vi "testBlockDMA_GERM.vi"(8 "error in (no error)":errorcluster, 11 "TestCase in":refnum<class "DSF CD GE Reflective Memory System Tests.lvclass">) -> (0 "error out":errorcluster, 3 "TestCase out":refnum<class "DSF CD GE Reflective Memory System Tests.lvclass">)   [LabVIEW 2019, in "DSF CD GE Reflective Memory System Tests.lvclass"]
uses:
  DSF CD GE Reflective Memory System Tests.lvclass
  C:/Program Files (x86)/National Instruments/LabVIEW 2019/vi.lib/addons/_JKI Toolkits/VI Tester/TestCase.llb/TestCase.lvclass
  niveristand-data-sharing-framework-custom-device-plugins/Components/Transceivers/GE Reflective Memory/Driver/Source/Typedefs/GE 5565PIORC.Typedef.DMA Wait Mode.ctl
  niveristand-data-sharing-framework-custom-device-plugins/Components/Transceivers/GE Reflective Memory/Driver/Source/GE 5565PIORC.lvclass
  <vilib>/addons/_JKI Toolkits/VI Tester/TestCase.llb/TestCase.lvclass
  fe7e187c-5126-4982-8e63-bd07b26320cd.vi
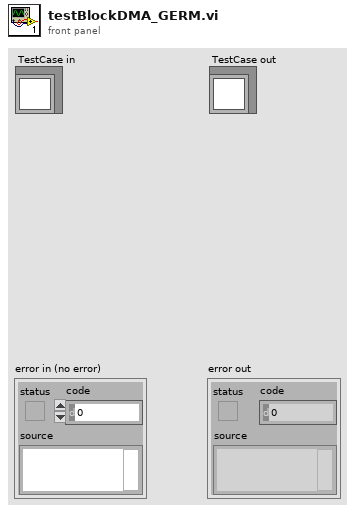
[diagram p1: front panel]
types:
  T1 = typedef "GE 5565PIORC.lvclass/GE 5565PIORC.Typedef.DMA Wait Mode.ctl" = enum16{"Polling", "Interrupt"}
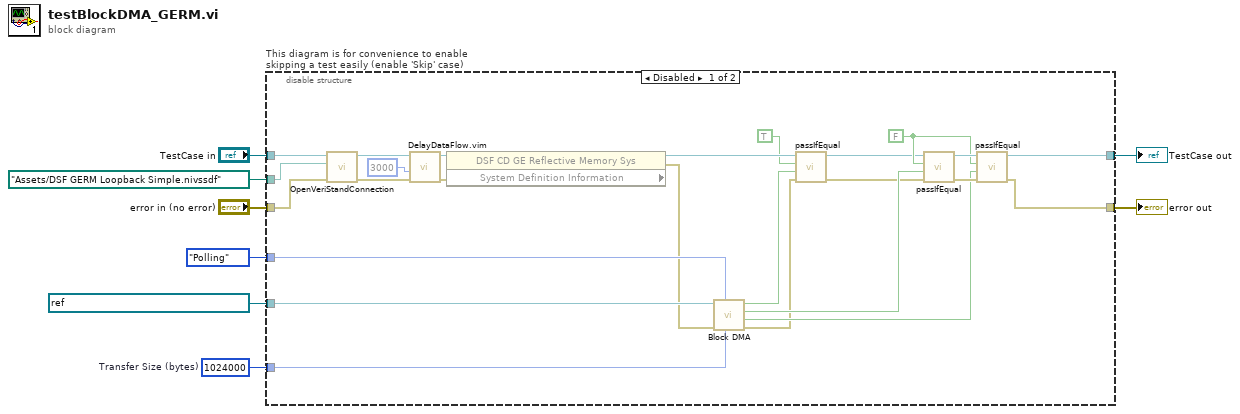
[diagram p0: block diagram]
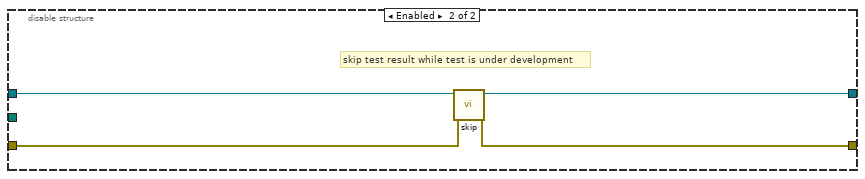
[diagram p2: hidden frame]
diagram:
  w2 = u32 1024000  # Transfer Size (bytes)
  n1 = disable-structure "This diagram is for convenience to enable skipping a test easily (enable 'Skip' case)" shown="Disabled" {
    disable-tunnel: "TestCase in" -> [w32 w36]
    disable-tunnel: [w29 w34] -> w7
    disable-tunnel: [w27 w35] -> w6
    disable-tunnel: "error in (no error)" -> [w25 w33]
    disable-tunnel: path "Assets/DSF GERM Loopback Simple.nivssdf" ("System Definition File") -> [w31 _]
    disable-tunnel: GE_5565PIORC.Typedef.DMA_Wait_Mode."Polling" ("Wait Mode") -> [w24 _]
    disable-tunnel: w2 -> [w21 _]
    disable-tunnel: refnum<visa-resource-name> "visa://10.2.109.77/PXI8::15::INSTR" ("VISA Resource Name") -> [w23 _]
    frame Disabled {
      w26 = FALSE ("timed out?")
      n2 = call-dynamic "OpenVeriStandConnection.vi"("error in (no error)"=w25, "System Definition File"=w31, "VeriStand Test Case in"=w32) -> ("error out"=w10:errorcluster, "VeriStand Test Case out"=w12:refnum<class "DSF CD GE Reflective Memory System Tests.lvclass">)  [unwired: 6 in, 1 out]
      n3 = call "DelayDataFlow.vim"("value in"=w10, "milliseconds to wait"=u32 3000) -> ("value out"=w9:errorcluster)  [unwired: 2 in, 1 out]
      n4 = property class="DSF CD GE Reflective Memory Sys" props=["System Definition Information"](reference=w12, error in=w9) -> (reference out=w19:refnum<class "DSF CD GE Reflective Memory System Tests.lvclass">, error out=w22:errorcluster)  [unwired: 1 out]
      n5 = call "Block DMA.vi"("Transfer Size (bytes)"=w21, "Wait Mode"=w24, "error in (no error)"=w22, "VISA Resource Name"=w23) -> ("error out"=w14:errorcluster, "Read Timed Out?"=w15:bool, "Write Timed Out?"=w20:bool, "Success?"=w16:bool)  [unwired: 4 in]
      n6 = call-dynamic "passIfEqual.vi"("error in (no error)"=w14, "y"=w16, "x"=TRUE ("timed out?"), "TestCase in"=w19) -> ("error out"=w13:errorcluster, "TestCase out"=w18:refnum<class "DSF CD GE Reflective Memory System Tests.lvclass">)  [unwired: 6 in]
      n7 = call-dynamic "passIfEqual.vi"("error in (no error)"=w13, "y"=w20, "x"=w26, "TestCase in"=w18) -> ("error out"=w28:errorcluster, "TestCase out"=w30:refnum<class "DSF CD GE Reflective Memory System Tests.lvclass">)  [unwired: 6 in]
      n8 = call-dynamic "passIfEqual.vi"("error in (no error)"=w28, "y"=w15, "x"=w26, "TestCase in"=w30) -> ("error out"=w27:errorcluster, "TestCase out"=w29:refnum<class "DSF CD GE Reflective Memory System Tests.lvclass">)  [unwired: 6 in]
    }
    frame Enabled {
      # "skip test result while test is under development"
      n9 = call <vilib>:"skip.vi"("error in (no error)"=w33, "TestCase in"=w36) -> ("error out"=w35:errorcluster, "TestCase out"=w34:refnum<class "DSF CD GE Reflective Memory System Tests.lvclass">)  [unwired: 8 in]
    }
  }
  "error out" <- w6
  "TestCase out" <- w7
